vi "Get Joystick 2015.vi"() -> (3 "Robot Controls":T1)   [LabVIEW 2014]
uses:
  Robot Control Outputs.ctl
  Global Variables/Refnum Names.vi
  <vilib>/Rock Robotics/WPI/Joystick/WPI_JoystickGetSetRefNum.vi
  <vilib>/Rock Robotics/Network Tables/SD Write Numeric Array.vi
  <vilib>/Rock Robotics/Network Tables/SD Write Boolean Array.vi
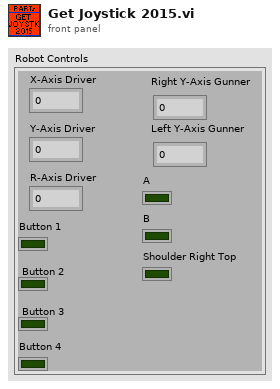
[diagram p1: front panel]
types:
  T1 = typedef "Robot Control Outputs.ctl" = cluster{"X-Axis Driver":dbl, "Y-Axis Driver":dbl, "R-Axis Driver":dbl, "Button 1":bool, "Button 2":bool, "Button 3":bool, "Button 4":bool, "Right Y-Axis Gunner":dbl, "Left Y-Axis Gunner":dbl, "A":bool, "B":bool, "Shoulder Right Top ":bool}
  T2 = typedef "WPI_JoystickDevRef.ctl" = cluster{"Device":T3}
  T3 = typedef "WPI_JoystickDeviceEnum.ctl" = enum16{"USB 0", "USB 1", "USB 2", "USB 3", "USB 4", "USB 5"}
  T4 = cluster{"Axes[0]":dbl, "Axes[1]":dbl, "Axes[2]":dbl, "Axes[3]":dbl, "Axes[4]":dbl, "Axes[5]":dbl, "Axes[6]":dbl, "Axes[7]":dbl, "Axes[8]":dbl}
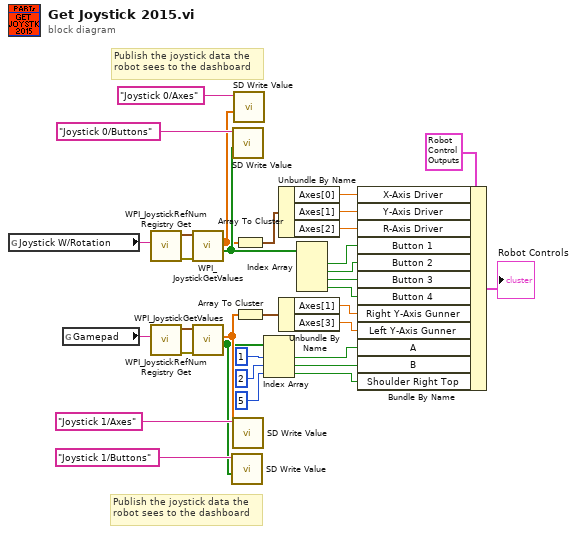
[diagram p0: block diagram]
diagram:
  # "Publish the joystick data the\nrobot sees to the dashboard"
  # "Publish the joystick data the\nrobot sees to the dashboard"
  n1 = global read "Refnum Names.vi" "Joystick W/Rotation"() -> (w31:string)
  n2 = global read "Refnum Names.vi" "Gamepad"() -> (w30:string)
  n3 = call <vilib>:"WPI_JoystickRefNum Registry Get.vi"("refnum name"=w31) -> ("error out"=w33:errorcluster, "JoystickDevRef"=w32:T2)  [unwired: 9 in]
  n4 = call <vilib>:"WPI_JoystickRefNum Registry Get.vi"("refnum name"=w30) -> ("error out"=w28:errorcluster, "JoystickDevRef"=w29:T2)  [unwired: 9 in]
  n5 = call <vilib>:"WPI_JoystickGetValues.vi"("error in (no error)"=w33, "JoystickDevRef"=w32) -> ("Buttons"=w8:bool[], "Axes"=w7:dbl[])  [unwired: 5 in, 3 out]
  n6 = call <vilib>:"WPI_JoystickGetValues.vi"("error in (no error)"=w28, "JoystickDevRef"=w29) -> ("Buttons"=w9:bool[], "Axes"=w10:dbl[])  [unwired: 5 in, 3 out]
  n7 = call-poly <vilib>:"SD Write Value.vi"("Boolean Array"=w9, "Name"="Joystick 1/Buttons") -> ()  [unwired: 8 in, 2 out]
  n8 = call-poly <vilib>:"SD Write Value.vi"("Boolean Array"=w8, "Name"="Joystick 0/Buttons") -> ()  [unwired: 8 in, 2 out]
  n9 = call-poly <vilib>:"SD Write Value.vi"("Numeric Array"=w10, "Name"="Joystick 1/Axes") -> ()  [unwired: 8 in, 2 out]
  n10 = call-poly <vilib>:"SD Write Value.vi"("Numeric Array"=w7, "Name"="Joystick 0/Axes") -> ()  [unwired: 8 in, 2 out]
  n11 = Array To Cluster(array=w7) -> (cluster=w27:T4)
  n12 = Array To Cluster(array=w10) -> (cluster=w26:T4)
  n13 = Index Array(array=w9, index #1=1 ("index"), index #2=2 ("index"), index #3=5 ("index")) -> (element #1=w4:bool, element #2=w5:bool, element #3=w6:bool)
  n14 = Unbundle By Name(w27) -> ("Axes[0]"=w25:dbl, "Axes[1]"=w24:dbl, "Axes[2]"=w23:dbl)
  n15 = Unbundle By Name(w26) -> ("Axes[1]"=w2:dbl, "Axes[3]"=w3:dbl)
  n16 = Index Array(array=w8) -> (element #1=w22:bool, element #2=w12:bool, element #3=w11:bool, element #4=w1:bool)  [unwired: 4 in]
  n17 = Bundle By Name(cluster=T1 {"X-Axis Driver"=0.0, "Y-Axis Driver"=0.0, "R-Axis Driver"=0.0, "Button 1"=FALSE, "Button 2"=FALSE, "Button 3"=FALSE, "Button 4"=FALSE, "Right Y-Axis Gunner"=0.0, "Left Y-Axis Gunner"=0.0, "A"=FALSE, "B"=FALSE, "Shoulder Right Top "=FALSE} ("Driver/Gunner Controls"), "X-Axis Driver"=w25, "Y-Axis Driver"=w24, "R-Axis Driver"=w23, "Button 1"=w22, "Button 2"=w12, "Button 3"=w11, "Button 4"=w1, "Right Y-Axis Gunner"=w2, "Left Y-Axis Gunner"=w3, "A"=w4, "B"=w5, "Shoulder Right Top"=w6) -> (→"Robot Controls":T1)
